vi "Simple_Тumbers.vi"() -> ()   [LabVIEW 2019]
panel:
  out "/Num":dbl
  in  "Number":dbl
  out "*Numbers":string
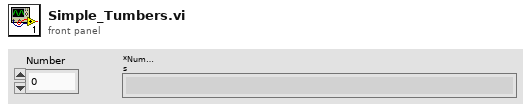
[diagram p1: front panel]
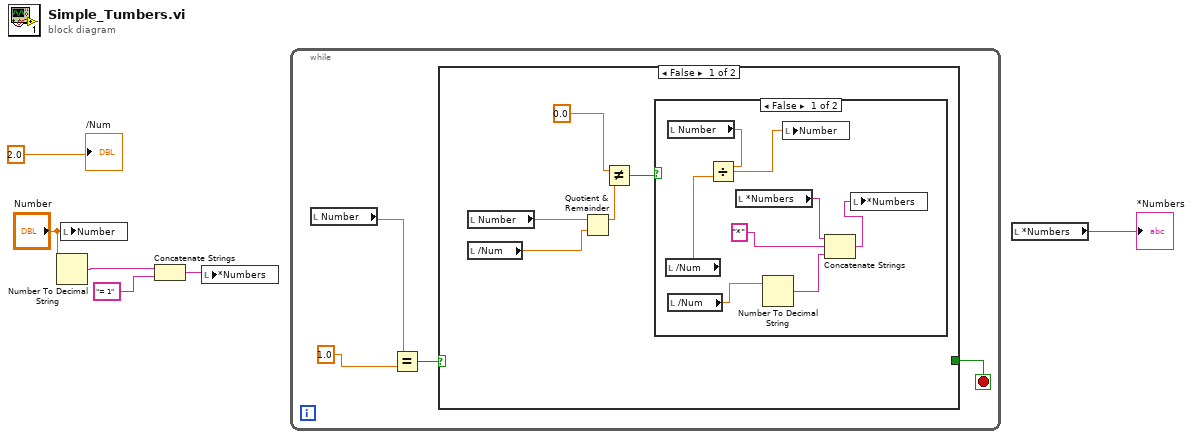
[diagram p0: block diagram]
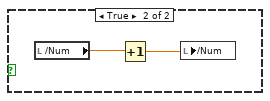
[diagram p2: hidden frame]
diagram:
  n1 = Number To Decimal String(number="Number") -> (decimal integer string=w4:string)  [unwired: 1 in]
  n2 = local write "Number"("Number") -> ()
  n3 = Concatenate Strings(w4, "= 1") -> (w5:string)
  n4 = local write "*Numbers"(w5) -> ()
  n5 = while {
    stop <- w8 stop-if-true
    n6 = local read "Number"() -> (w10:dbl)
    n7 = Equal?(x=w10, y=1.0 ("Number")) -> (x = y?=w9:bool)
    n8 = case shown="False" w9 {
      selector: w9 -> [_ w26]
      tunnel: [_ w26] -> w8
      frame False {
        n9 = local read "Number"() -> (w15:dbl)
        n10 = local read "/Num"() -> (w14:dbl)
        n11 = Quotient & Remainder(x=w15, y=w14) -> (x-y*floor(x/y)=w12:dbl)  [unwired: 1 out]
        n12 = Not Equal?(x=0.0 ("Number"), y=w12) -> (x != y?=w13:bool)
        n13 = case shown="False" w13 {
          frame False {
            n14 = local read "/Num"() -> (w21:dbl)
            n15 = local read "Number"() -> (w23:dbl)
            n16 = local read "/Num"() -> (w17:dbl)
            n17 = Divide(x=w23, y=w21) -> (x/y=w22:dbl)
            n18 = local read "*Numbers"() -> (w20:string)
            n19 = Number To Decimal String(number=w17) -> (decimal integer string=w16:string)  [unwired: 1 in]
            n20 = local write "Number"(w22) -> ()
            n21 = Concatenate Strings(w20, "*", w16) -> (w18:string)
            n22 = local write "*Numbers"(w18) -> ()
          }
          frame True {
            n23 = local read "/Num"() -> (w25:dbl)
            n24 = Increment(x=w25) -> (x+1=w24:dbl)
            n25 = local write "/Num"(w24) -> ()
          }
        }
      }
      frame True {
      }
    }
  }
  n26 = local read "*Numbers"() -> (→"*Numbers":string)
  "/Num" <- 2.0
